vi "字符变换.vi"(1 "替换字符串数组":string[][](array[string])=[["#$%01%$#", "HZHEHUA"], ["#$%02%$#", "12345678"], ["#$%03%$#", "ABCDE"], ["#$%04%$#", "杭州和华2018年"]], 2 "输入字符串":string="^XA~TA000~JSN^LT0^MNW^MTT^PON^PMN^LH0,0^JMA^PR5,5~SD20^JUS^LRN^CI0^XZ\n~DG000.GRF,00768,012,\n,::::::::::::::::::::::P020,K0IFE0208FF8,K0IFE020C7F0,K080020FFE618,K080030FFE410,K080020208E18,K0C002020C410,K0800203F8FF8C0,K0800203F87F0C0,K080020208E18C0,K0IFE020C410,K0IFE03F8E18,K0800303F8410,K080020208FF8,K0C002020C7F0,K080020FFEC18,K080020FFE41040,K080020108818E0,K0C0020118C10C0,K0IFE060C838,K0JF0C011F0,K0800208038E0,K0C0020,,:::::::::::::::::^XA\n^MMT\n^PW320\n^LL0240\n^LS0\n^FT0,128^XG000.GRF,1,1^FS\n^FT16,50^A0N,34,33^FH\\^FD#$%01%$#^FS\n^BY2,3,61^FT40,189^BCN,,Y,N\n^FD>:#$%02%$#^FS\n^FT200,136^BQN,2,5\n^FH\\^FDLA,#$%03%$#^FS\n^FT72,103^A0N,23,24^FH\\^FD#$%04%$#^FS\n^PQ1,0,1,Y^XZ\n^XA^ID000.GRF^FS^XZ\n") -> (0 "输出字符串":string)   [LabVIEW 2018]
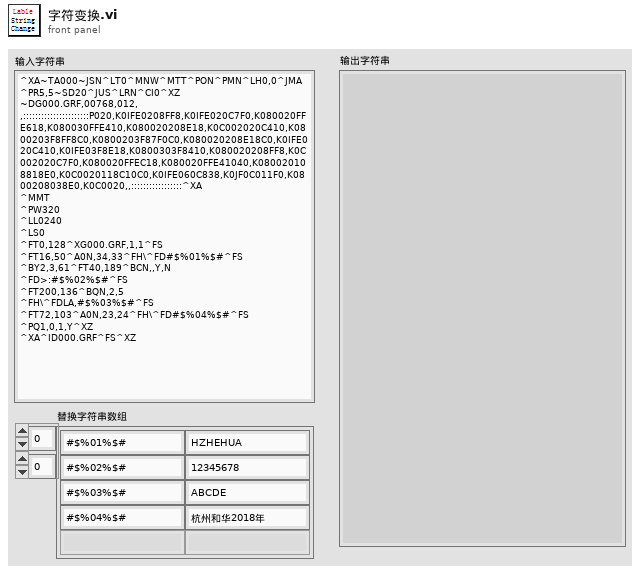
[diagram p1: front panel]
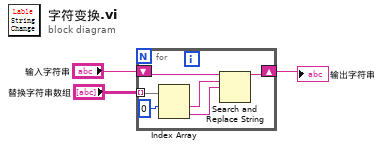
[diagram p0: block diagram]
diagram:
  n1 = for {
    tunnel: "替换字符串数组" -> [w9] mode=indexing
    shift-right: [w6] -> w2
    shift-left: "输入字符串" -> [w7]
    n2 = Index Array(array=w9, index #1=0 ("索引")) -> (element #1=w5:string, element #2=w4:string)  [unwired: 1 in]
    n3 = Search and Replace String(input string=w7, search string=w5, replace string=w4) -> (result string=w6:string)  [unwired: 5 in, 3 out]
  }
  "输出字符串" <- w2
